vi "B Spoof Relative Wind.vi"(6 "Wind Speed":dbl, 7 "Wind Angle":T3 format="%05.1f", 8 "Velocity (3 array)":dbl[](array[numeric])) -> (0 "Apparent Wind\nSpeed":T1, 1 "Perceived Wind":cluster{"X Position":dbl, "Y Position":dbl}, 2 "Apparent Wind\nDirection":T2, 3 "Global Wind":cluster{"X Position":dbl, "Y Position":dbl}, 5 "Robot\nHeading":T3 format="%05.1f")   [LabVIEW 2011]
uses:
  2-Think/2 Typedefs/heading.ctl
  2-Think/2 Typedefs/apparent wind direction.ctl
  2-Think/2 Typedefs/apparent wind speed.ctl
  <vilib>/Analysis/_algsub.llb/Real Vector Norm.vi
  <vilib>/Analysis/baseanly.llb/Real Dot Product.vi
  <vilib>/Analysis/NI_AALPro.lvlib
  <vilib>/Analysis/NI_AALBase.lvlib
panel:
  out "Heading unit\nvector":cluster{"X Position":dbl, "Y Position":dbl}
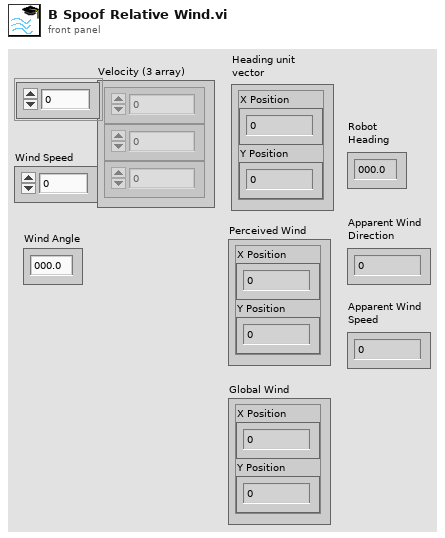
[diagram p1: front panel]
types:
  T1 = typedef "apparent wind speed.ctl" = dbl
  T2 = typedef "apparent wind direction.ctl" = dbl
  T3 = typedef "heading.ctl" = dbl
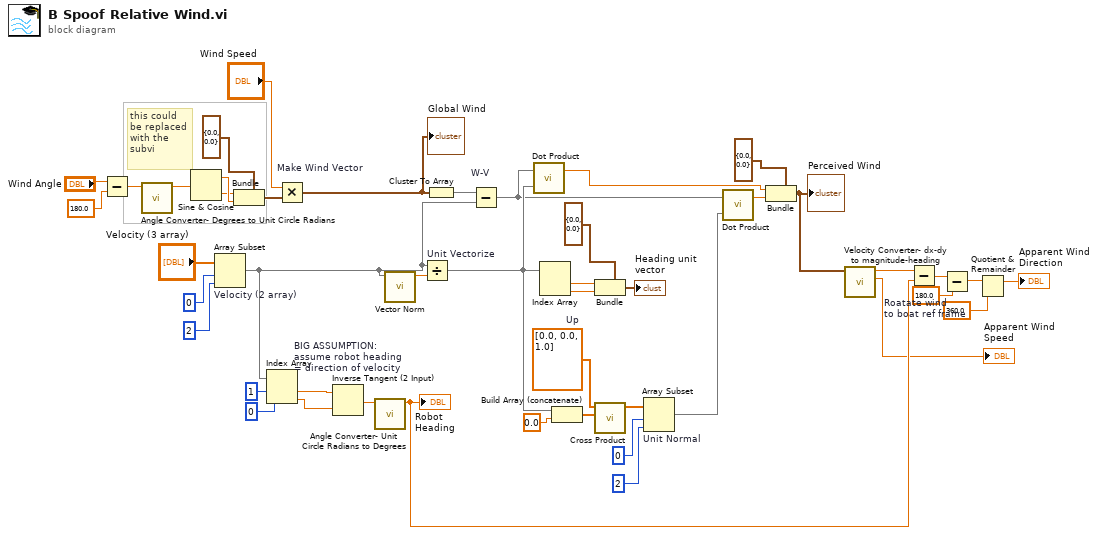
[diagram p0: block diagram]
diagram:
  w20 = dbl[] [0.0, 0.0, 1.0]  # Up
  # "this could\nbe replaced\nwith the\nsubvi"
  n1 = Subtract(x="Wind Angle", y=T3 180.0 ("Wind Angle 2")) -> (x-y=w18:T3)
  n2 = call "Angle Converter- Degrees to Unit Circle Radians.vi"("Angle in \nHeading \nFormat"=w18) -> ("Angle in \nUnit Circle\nRadians"=w19:dbl)  [unwired: 10 in]
  n3 = Sine & Cosine(0:w19) -> (1:w34:dbl, 2:w33:dbl)
  n4 = Array Subset "Velocity (2 array)"(array="Velocity (3 array)", index=0, length=2) -> (w12:dbl[])
  n5 = Bundle(cluster=cluster{"X Position":dbl, "Y Position":dbl} {"X Position"=0.0, "Y Position"=0.0} ("Robot Location"), "X Position"=w33, "Y Position"=w34) -> (w35:cluster{"X Position":dbl, "Y Position":dbl})
  n6 = Index Array(array=w12, index #1=1 ("index"), index #2=0 ("index")) -> (element #1=w14:dbl, element #2=w13:dbl)
  n7 = Multiply "Make Wind Vector"(x="Wind Speed", y=w35) -> (x*y=w38:cluster{"X Position":dbl, "Y Position":dbl})
  "Global Wind" <- w38
  n8 = Inverse Tangent (2 Input) "BIG ASSUMPTION:\nassume robot heading\n= direction of velocity"(1:w13, 2:w14) -> (0:w15:dbl)
  n9 = call "Angle Converter- Unit Circle Radians to Degrees.vi"("Angle in \nUnit Circle\nRadians"=w15) -> ("Angle in \nHeading \nFormat"=w5:T3)  [unwired: 10 in]
  "Robot\nHeading" <- w5
  n10 = call-poly <vilib>:"Vector Norm.vi"("Input Vector"=w12) -> ("norm"=w46:dbl)  [unwired: 9 in, 1 out]
  n11 = Divide "Unit Vectorize"(x=w12, y=w46) -> (x/y=w29:dbl[])
  n12 = Cluster To Array(cluster=w38) -> (array=w43:dbl[])
  n13 = Subtract "W-V"(x=w43, y=w12) -> (x-y=w24:dbl[])
  n14 = call-poly <vilib>:"Dot Product.vi"("Y Vector"=w29, "X Vector"=w24) -> ("X * Y"=w45:dbl)  [unwired: 1 out]
  n15 = Index Array(array=w29) -> (element #1=w40:dbl, element #2=w41:dbl)  [unwired: 2 in]
  n16 = Build Array (concatenate)(w29, 0.0) -> (w21:dbl[])
  n17 = Bundle(cluster=cluster{"X Position":dbl, "Y Position":dbl} {"X Position"=0.0, "Y Position"=0.0} ("Robot Location"), "X Position"=w40, "Y Position"=w41) -> (→"Heading unit\nvector":cluster{"X Position":dbl, "Y Position":dbl})
  n18 = call <vilib>:"Cross Product.vi"("B Vector"=w21, "A Vector"=w20) -> ("Cross Product"=w25:dbl[])  [unwired: 8 in, 1 out]
  n19 = Array Subset "Unit Normal"(array=w25, index=0, length=2) -> (w23:dbl[])
  n20 = call-poly <vilib>:"Dot Product.vi"("Y Vector"=w23, "X Vector"=w24) -> ("X * Y"=w22:dbl)  [unwired: 1 out]
  n21 = Bundle(cluster=cluster{"X Position":dbl, "Y Position":dbl} {"X Position"=0.0, "Y Position"=0.0} ("Perceived Wind"), "X Position"=w45, "Y Position"=w22) -> (w7:cluster{"X Position":dbl, "Y Position":dbl})
  "Perceived Wind" <- w7
  n22 = call "Velocity Converter- dx-dy to magnitude-heading.vi"("Vector In"=w7) -> ("Magnitude Out"=→"Apparent Wind\nSpeed":dbl, "Heading Out"=w6:T3)  [unwired: 9 in]
  n23 = Subtract "Roatate wind\nto boat ref frame"(x=w6, y=w5) -> (x-y=w9:T3)
  n24 = Subtract(x=w9, y=T3 180.0) -> (x-y=w3:T3)
  n25 = Quotient & Remainder(x=w3, y=T3 360.0) -> (x-y*floor(x/y)=→"Apparent Wind\nDirection":T3)  [unwired: 1 out]
